vi "RPT_Report Generate.vi"(8 "Report Name":string="Test_1", 9 "template":path=path "M:/OLS Level Test Project/PWC-OLS/$ReportFiles/ReportTemplate_01.xlsx", 10 "Results":T1=[[{"Fill"=0.0, "Drain"=7.612782182151588, "Status"=5, "Resistor"=100.2}, {"Fill"=3.699999999999991, "Drain"=7.368700152811735, "Status"=9, "Resistor"=100.4}], [{"Fill"=7.519750916870415, "Drain"=7.144624847188264, "Status"=5, "Resistor"=199.3}, {"Fill"=7.323685024449877, "Drain"=6.908545507334963, "Status"=5, "Resistor"=199.4}], [{"Fill"=7.101610391198044, "Drain"=6.69747457212714, "Status"=5, "Resistor"=298.5}, {"Fill"=6.859529034229828, "Drain"=6.46039489608802, "Status"=5, "Resistor"=298.4}], [{"Fill"=6.616447341075794, "Drain"=6.23331858190709, "Status"=5, "Resistor"=397.6}, {"Fill"=6.4163801039119805, "Drain"=6.007242603911981, "Status"=5, "Resistor"=397.6}], [{"Fill"=6.176299419315403, "Drain"=5.775164608801956, "Status"=5, "Resistor"=497.4}, {"Fill"=5.938219407090465, "Drain"=5.544086949877751, "Status"=5, "Resistor"=497.2}], [{"Fill"=5.733150488997555, "Drain"=5.331015342298288, "Status"=5, "Resistor"=597.7}, {"Fill"=5.478064761613692, "Drain"=5.0889339853300735, "Status"=5, "Resistor"=597.0}], [{"Fill"=5.25498979217604, "Drain"=4.853854981662591, "Status"=5, "Resistor"=697.7}, {"Fill"=5.02791347799511, "Drain"=4.634781356968215, "Status"=5, "Resistor"=697.0}], [{"Fill"=4.795835482885085, "Drain"=4.415707732273838, "Status"=5, "Resistor"=797.9}, {"Fill"=4.572760513447433, "Drain"=0.0, "Status"=5, "Resistor"=797.2}], [{"Fill"=4.368691931540343, "Drain"=3.9545527506112466, "Status"=5, "Resistor"=897.6}, {"Fill"=4.125610238386308, "Drain"=4.172626039119804, "Status"=10, "Resistor"=856.6}], [{"Fill"=3.90853728606357, "Drain"=0.0, "Status"=5, "Resistor"=998.1}, {"Fill"=3.68246130806846, "Drain"=3.7114710574572127, "Status"=10, "Resistor"=897.1}], [{"Fill"=3.45638533007335, "Drain"=3.389362805623472, "Status"=10, "Resistor"=998.3}, {"Fill"=3.200299266503668, "Drain"=3.010235391198044, "Status"=10, "Resistor"=997.4}]] {"Resistor" format="%.1f"; "Drain" format="%.3f"; "Fill" format="%.3f"}, 11 "Wave Data":dbl[][](array[numeric])=array12946x5[64730 elements]) -> ()   [LabVIEW 2024]
uses:
  Control Definitions/Def Results2.ctl
  <vilib>/Utility/NIReport.llb/Report Type.ctl
  <vilib>/addons/_office/excel.llb/Excel Easy Table (str).vi
  <vilib>/Utility/NIReport.llb/NI_report.lvclass
  <vilib>/Utility/NIReport.llb/NI_ReportGenerationCore.lvlib
  <vilib>/Utility/NIReport.llb/Excel/NI_Excel.lvclass
  <vilib>/addons/_office/NI_ReportGenerationToolkit.lvlib
panel:
  out "Results size":i32[](array[numeric])
  out "Wave Data size":i32[](array[numeric])
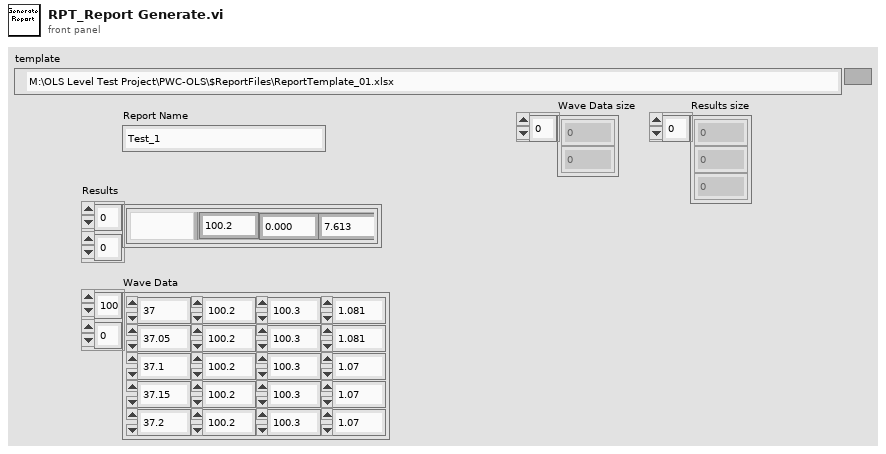
[diagram p1: front panel]
types:
  T1 = typedef "Def Results2.ctl" = cluster{"Fill":dbl, "Drain":dbl, "Status":i16, "Resistor":dbl}[][]
  T2 = typedef "NI_ReportGenerationCore.lvlib/Report Type.ctl" = enum16{"HTML", "Word", "Excel"}
  T3 = cluster{"left":i32, "top":i32, "height":dbl, "width":dbl}
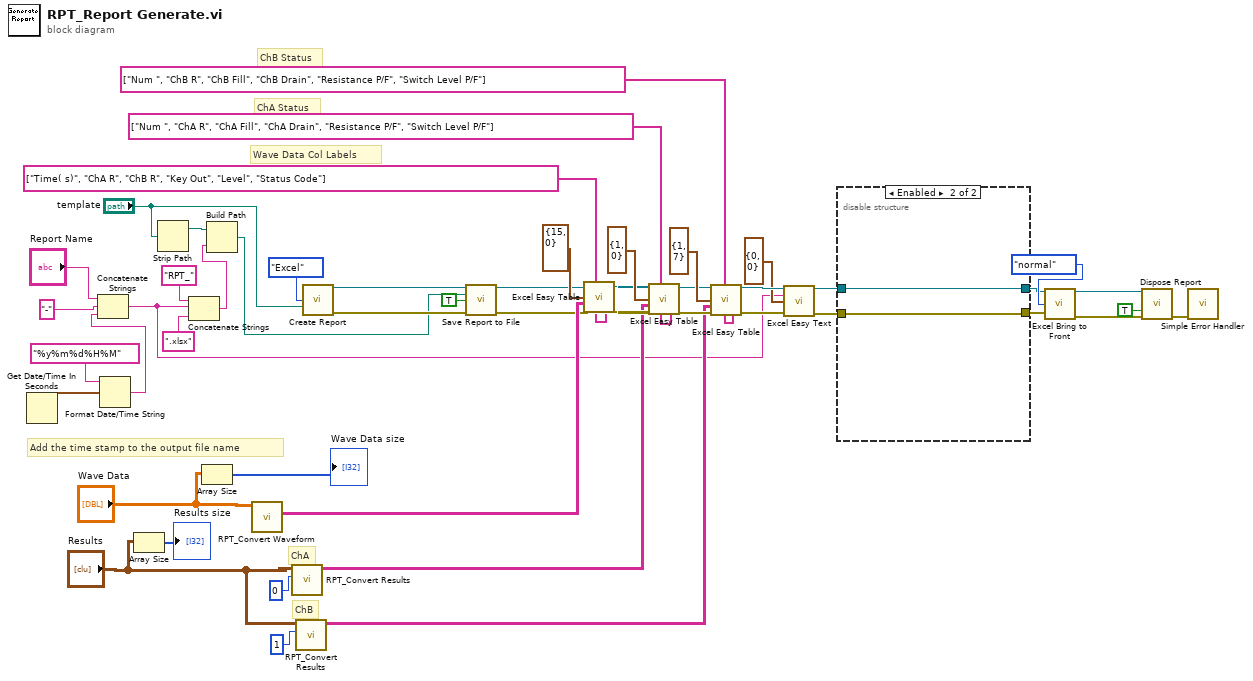
[diagram p0: block diagram]
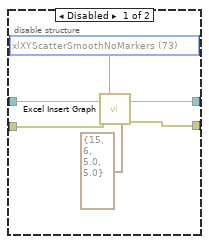
[diagram p2: hidden frame]
diagram:
  # "Add the time stamp to the output file name"
  # "ChB Status"
  # "ChA Status"
  # "Wave Data Col Labels"
  # "ChB"
  # "ChA"
  n1 = Get Date/Time In Seconds() -> (seconds since 1Jan1904=w15:timestamp)
  n2 = Format Date/Time String(time format string (%c)="%y%m%d%H%M", seconds (now)=w15) -> (date/time string=w16:string)  [unwired: 1 in]
  n3 = Concatenate Strings("Report Name", "-" ("string"), w16) -> (w5:string)
  n4 = Array Size(array="Results") -> (size(s)=→"Results size":i32[])
  n5 = Strip Path(path="template") -> (stripped path=w25:path)  [unwired: 1 out]
  n6 = Concatenate Strings("RPT_", w5, ".xlsx") -> (w6:string)
  n7 = Array Size(array="Wave Data") -> (size(s)=→"Wave Data size":i32[])
  n8 = Build Path(base path=w25, name or relative path=w6) -> (appended path=w20:path)
  n9 = call "RPT_Convert Waveform.vi"("Wave Data IN"="Wave Data") -> ("Text OUT"=w44:string[][])  [unwired: 8 in, 2 out]
  n10 = call "RPT_Convert Results.vi"("disabled index (col)"=0, "Results IN"="Results") -> ("Report OUt"=w31:string[][])  [unwired: 9 in]
  n11 = call "RPT_Convert Results.vi"("disabled index (col)"=1, "Results IN"="Results") -> ("Report OUt"=w29:string[][])  [unwired: 9 in]
  n12 = call <vilib>:"Create Report.vi"("report type"=Report_Type."Excel" ("Report Type"), "template (empty)"="template") -> ("report out"=w24:refnum<class "NI_report.lvclass">, "error out"=w21:errorcluster)  [unwired: 12 in]
  n13 = call-dynamic "Save Report to File.vi"("report in"=w24, "report file path"=w20, "prompt to replace? (F)"=TRUE, "error in (no error)"=w21) -> ("report out"=w23:refnum<class "NI_report.lvclass">, "error out"=w22:errorcluster)  [unwired: 10 in]
  n14 = call-poly <vilib>:"Excel Easy Table.vi"("report in"=w23, "start (0, 0)"=cluster{"row":i32, "column":i32} {"row"=15, "column"=0}, "text data"=w44, "error in (no error)"=w22, "column headers"=string[] ["Time( s)", "ChA R", "ChB R", "Key Out", "Level", "Status Code"]) -> ("report out"=w38:refnum<class "NI_report.lvclass">, "error out"=w37:errorcluster)  [unwired: 6 in, 3 out]
  n15 = call-poly <vilib>:"Excel Easy Table.vi"("report in"=w38, "start (0, 0)"=cluster{"row":i32, "column":i32} {"row"=1, "column"=0}, "text data"=w31, "error in (no error)"=w37, "column headers"=string[] ["Num ", "ChA R", "ChA Fill", "ChA Drain", "Resistance P/F", "Switch Level P/F"]) -> ("report out"=w40:refnum<class "NI_report.lvclass">, "error out"=w39:errorcluster)  [unwired: 6 in, 3 out]
  n16 = call-poly <vilib>:"Excel Easy Table.vi"("report in"=w40, "start (0, 0)"=cluster{"row":i32, "column":i32} {"row"=1, "column"=7}, "text data"=w29, "error in (no error)"=w39, "column headers"=string[] ["Num ", "ChB R", "ChB Fill", "ChB Drain", "Resistance P/F", "Switch Level P/F"]) -> ("report out"=w12:refnum<class "NI_report.lvclass">, "error out"=w11:errorcluster)  [unwired: 6 in, 3 out]
  n17 = call <vilib>:"Excel Easy Text.vi"("report in"=w12, "text"=w5, "start (-1, -1)"=cluster{"row":i32, "column":i32} {"row"=0, "column"=0}, "error in (no error)"=w11) -> ("report out"=w14:refnum<class "NI_report.lvclass">, "error out"=w13:errorcluster)  [unwired: 7 in, 3 out]
  n18 = disable-structure shown="Enabled" {
    disable-tunnel: w14 -> [w53 w57]
    disable-tunnel: w13 -> [w52 w56]
    disable-tunnel: [w51 w56] -> w33
    disable-tunnel: [w50 w57] -> w32
    frame Disabled {
      w54 = 73 items=["xlColumnClustered"=51, "xlColumnStacked"=52, "xlColumnStacked100"=53, "xl3DColumnClustered"=54, "xl3DColumnStacked"=55, "xl3DColumnStacked100"=56, "xlBarClustered"=57, "xlBarStacked"=58, "xlBarStacked100"=59, "xl3DBarClustered"=60, "xl3DBarStacked"=61, "xl3DBarStacked100"=62, "xlLineStacked"=63, "xlLineStacked100"=64, "xlLineMarkers"=65, "xlLineMarkersStacked"=66, "xlLineMarkersStacked100"=67, "xlPieOfPie"=68, "xlPieExploded"=69, "xl3DPieExploded"=70, "xlBarOfPie"=71, "xlXYScatterSmooth"=72, "xlXYScatterSmoothNoMarkers"=73, "xlXYScatterLines"=74, "xlXYScatterLinesNoMarkers"=75, "xlAreaStacked"=76, "xlAreaStacked100"=77, "xl3DAreaStacked"=78, "xl3DAreaStacked100"=79, "xlDoughnutExploded"=80, "xlRadarMarkers"=81, "xlRadarFilled"=82, "xlSurface"=83, "xlSurfaceWireframe"=84, "xlSurfaceTopView"=85, "xlSurfaceTopViewWireframe"=86, "xlBubble"=15, "xlBubble3DEffect"=87, "xlStockHLC"=88, "xlStockOHLC"=89, "xlStockVHLC"=90, "xlStockVOHLC"=91, "xlCylinderColClustered"=92, "xlCylinderColStacked"=93, "xlCylinderColStacked100"=94, "xlCylinderBarClustered"=95, "xlCylinderBarStacked"=96, "xlCylinderBarStacked100"=97, "xlCylinderCol"=98, "xlConeColClustered"=99, "xlConeColStacked"=100, "xlConeColStacked100"=101, "xlConeBarClustered"=102, "xlConeBarStacked"=103, "xlConeBarStacked100"=104, "xlConeCol"=105, "xlPyramidColClustered"=106, "xlPyramidColStacked"=107, "xlPyramidColStacked100"=108, "xlPyramidBarClustered"=109, "xlPyramidBarStacked"=110, "xlPyramidBarStacked100"=111, "xlPyramidCol"=112, "xl3DColumn"=-4100, "xlLine"=4, "xl3DLine"=-4101, "xl3DPie"=-4102, "xlPie"=5, "xlXYScatter"=-4169, "xl3DArea"=-4098, "xlArea"=1, "xlDoughnut"=-4120, "xlRadar"=-4151] ("chart type")
      n19 = call <vilib>:"Excel Insert Graph.vi"("report in"=w53, "graph type (col clustered)"=w54, "error in (no error)"=w52, "position/size"=T3 {"left"=15, "top"=6, "height"=5.0, "width"=5.0}) -> ("report out"=w50:refnum<class "NI_report.lvclass">, "error out"=w51:errorcluster)  [unwired: 10 in]
    }
    frame Enabled {
    }
  }
  n20 = call <vilib>:"Excel Bring to Front.vi"("report in"=w32, "window state (maximized)"=enum16{"maximized", "minimized", "normal"}."normal", "error in (no error)"=w33) -> ("report out"=w46:refnum<class "NI_report.lvclass">, "error out"=w47:errorcluster)  [unwired: 11 in]
  n21 = call-dynamic "Dispose Report.vi"("report in"=w46, "save changes? (F)"=TRUE, "error in (no error)"=w47) -> ("error out"=w45:errorcluster)  [unwired: 12 in]
  n22 = call <vilib>:"Simple Error Handler.vi"("error in (no error)"=w45) -> ()  [unwired: 4 in, 5 out]
